vi "Init DAQmx Event.vi"(8 "error in (no error)":errorcluster, 11 "DAQmxDI in":refnum<class "DAQmxDI.lvclass">) -> (0 "error out":errorcluster, 3 "DAQmxDI out":refnum<class "DAQmxDI.lvclass">, 4 "Event Reg":refnum<event-registration>)   [LabVIEW 2020, in "VolatusDAQ.lvlib" / "DAQmxDI.lvclass"]
uses:
  DAQmxDI.lvclass
  DAQmxDI.lvclass/DAQmxDI.ctl
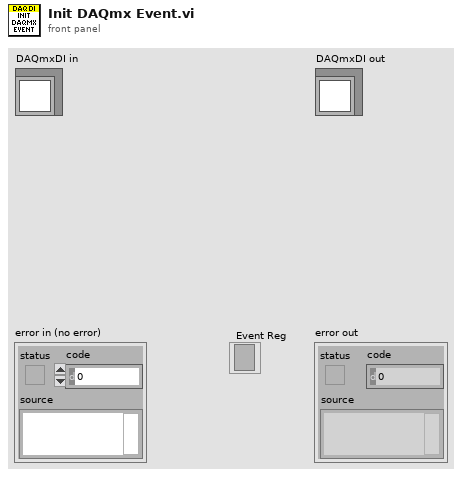
[diagram p1: front panel]
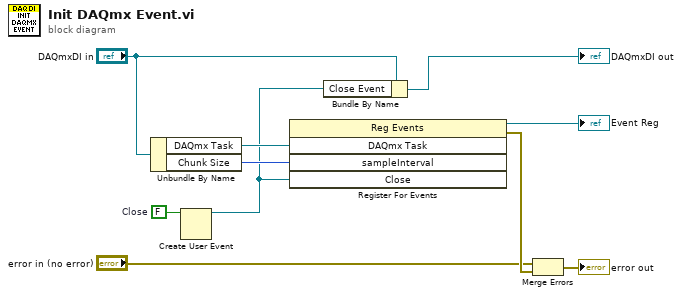
[diagram p0: block diagram]
diagram:
  w8 = FALSE  # Close
  n1 = Unbundle By Name("DAQmxDI in") -> ("DAQmx Task"=w10:refnum<k21>, "Chunk Size"=w9:i32)
  n2 = Create User Event(user event datatype=w8) -> (user event=w1:refnum<user-event>)  [unwired: 1 in, 1 out]
  n3 = register-events(w10, w9, w1) -> (reference out=→"Event Reg":refnum<event-registration>, error out=w6:errorcluster)  [unwired: 2 in]
  n4 = Bundle By Name(cluster="DAQmxDI in", "Close Event"=w1) -> (→"DAQmxDI out":refnum<class "DAQmxDI.lvclass">)
  n5 = Merge Errors("error in (no error)", w6) -> (→"error out":errorcluster)
